vi "VHMI-recieveData.vi"(8 "error in (no error)":errorcluster, 10 "VNA data":T1, 11 "VDH-VNA_data_handler in":refnum<class "VDH-VNA_data_handler.lvclass">) -> (0 "error out":errorcluster, 3 "VDH-VNA_data_handler out":refnum<class "VDH-VNA_data_handler.lvclass">)   [LabVIEW 2020, in "VDH-VNA_data_handler.lvlib" / "VDH-VNA_data_handler.lvclass"]
uses:
  VDH-VNA_data_handler.lvclass
  classes/vna-drivers/liteVNA/VD-VNA_data.ctl
  VDH-VNA_data_handler.lvclass/VDH-VNA_data_handler.ctl
  VDHI-VNA_data_handler_interface Messages/VHDI-recieveData Msg/VHDI-recieveData Msg.lvclass/VHDI-recieveData Msg.ctl
  <vilib>/ActorFramework/Message Enqueuer/Message Enqueuer.lvclass/Message Enqueuer.ctl
  <vilib>/ActorFramework/Message Enqueuer/Enqueue.vi
  VDHI-VNA_data_handler_interface Messages/VHDI-recieveData Msg/VHDI-recieveData Msg.lvclass
  C:/Program Files (x86)/National Instruments/LabVIEW 2020/vi.lib/ActorFramework/Message/Message.lvclass
  <vilib>/ActorFramework/Message Priority Queue/Priority Enqueue.vi
  classes/vna-drivers/liteVNA/VD-LV-LiteVNA.lvclass
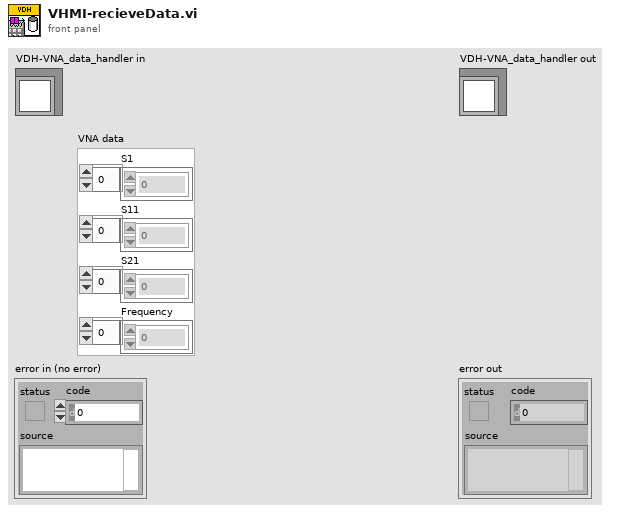
[diagram p1: front panel]
types:
  T1 = typedef "VD-LV-LiteVNA.lvclass/VD-VNA_data.ctl" = cluster{"S1":cdb[], "S11":cdb[], "S21":cdb[], "Frequency":u64[]}
  T2 = typedef "VDH-VNA_data_handler.lvlib/VDH-VNA_data_handler.lvclass/VDH-VNA_data.ctl" = cluster{"RP1":dbl[], "IP1":dbl[], "RP11":dbl[], "IP11":dbl[], "RP21":dbl[], "IP21":dbl[], "Frequency":u64[]}
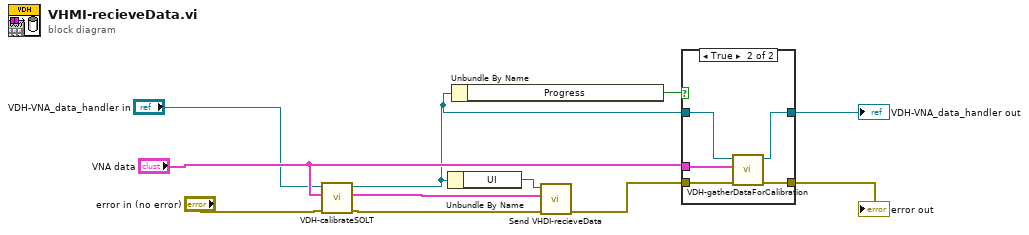
[diagram p0: block diagram]
diagram:
  n1 = call "VDH-calibrateSOLT.vi"("error in (no error)"="error in (no error)", "VNA data"="VNA data", "VDH-VNA_data_handler in"="VDH-VNA_data_handler in") -> ("error out"=w2:errorcluster, "output cluster"=w1:T2, "VDH-VNA_data_handler out"=w4:refnum<class "VDH-VNA_data_handler.lvclass">)  [unwired: 6 in]
  n2 = Unbundle By Name(w4) -> ("UI"=w11:refnum<class "Message Enqueuer.lvclass">)
  n3 = Unbundle By Name(w4) -> ("Progress"=w8:bool)
  n4 = call "Send VHDI-recieveData.vi"("error in (no error)"=w2, "Data"=w1, "Message Enqueuer"=w11) -> ("error out"=w10:errorcluster)  [unwired: 7 in, 1 out]
  n5 = case shown="True" w8 {
    tunnel: w4 -> [w12 w16]
    tunnel: w10 -> [w13 w18]
    tunnel: [w13 w17] -> w9
    tunnel: [w12 w15] -> w7
    tunnel: "VNA data" -> [_ w14]
    frame False {
    }
    frame True {
      n6 = call "VDH-gatherDataForCalibration.vi"("error in (no error)"=w18, "VNA data"=w14, "VDH-VNA_data_handler in"=w16) -> ("error out"=w17:errorcluster, "VDH-VNA_data_handler out"=w15:refnum<class "VDH-VNA_data_handler.lvclass">)  [unwired: 7 in]
    }
  }
  "error out" <- w9
  "VDH-VNA_data_handler out" <- w7
